vi "CB Make LQR Cost Matrix.vi"(11 "q":dbl[](array[numeric]) format="%.2f") -> (3 "Q":T1)   [LabVIEW 2020]
uses:
  <vilib>/Analysis/Matrix/Datatypes/RealMatrix.ctl
  <vilib>/Analysis/7linalg.llb/Create Special Real Matrix.vi
  <vilib>/Analysis/NI_AALPro.lvlib
  <vilib>/Analysis/Matrix/NI_Matrix.lvlib
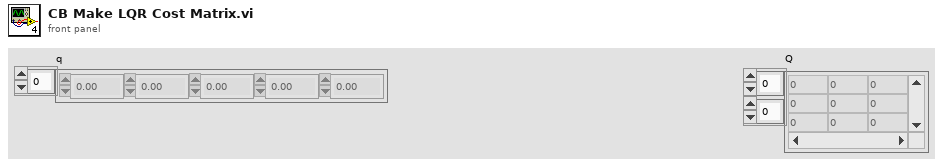
[diagram p1: front panel]
types:
  T1 = typedef "NI_Matrix.lvlib/RealMatrix.ctl" = dbl[][]
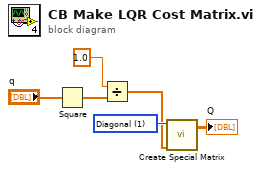
[diagram p0: block diagram]
diagram:
  w6 = 1 items=["Identity", "Diagonal", "Toeplitz", "Vandermonde", "Companion", "Hankel", "Hadamard", "Wilkinson", "Hilbert", "Inverse Hilbert", "Rosser", "Pascal"] ("matrix type")
  n1 = Square(x="q") -> (x^2=w4:dbl[])
  n2 = Divide(x=1.0, y=w4) -> (x/y=w2:dbl[])
  n3 = call-poly <vilib>:"Create Special Matrix.vi"("matrix type"=w6, "Input Vector1"=w2) -> ("Special Matrix"=→"Q":T1)  [unwired: 3 in, 1 out]
